vi "FFT.vi"() -> ()   [LabVIEW 2020]
uses:
  <vilib>/rvi/Analysis/measure/FFT/simModelSupport/niFPGA FFT Outside SCTL Sim Properties.ctl
  <vilib>/rvi/Analysis/measure/FFT/simModelSupport/niFPGA FFT Sim Types.ctl
  <vilib>/rvi/Analysis/measure/FFT/simModelSupport/niFpgaFFTSimArithmeticProperties.ctl
  <vilib>/rvi/Analysis/measure/FFT/simModelSupport/niFpgaFFTSimDfxp.ctl
  <vilib>/fxp/LVFixedPointQuantizationPolicyTypeDef.ctl
  <vilib>/rvi/Emulation/niFpgaGetClockAttributes.vi
  <vilib>/rvi/Emulation/niFpgaSctlEmulationGetInTimedLoop.vi
  <vilib>/rvi/Emulation/niFpgaEmulationReportErrorSimple.vi
  <vilib>/rvi/interface/RandomDataEmulation/niFpgaRandomDataHandleErrors.vi
  <vilib>/rvi/Analysis/measure/FFT/simModelSupport/niFpgaFFTSimModelOutsideSCTLCore.vi
  <vilib>/rvi/Emulation/niFpgaCriticalErrorInLSC.vi
  <vilib>/rvi/DataTransferAndStorage/Container/XNode/niFpgaContainer.xnode
  <vilib>/rvi/interface/RandomDataEmulation/nirviRandomDataFpgaReadWriteTemplate.vi
  <vilib>/rvi/Analysis/measure/FFT/XNode/niFpgaFFT.xnode
panel:
  out "x-y (microsecond)":u32
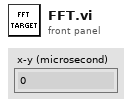
[diagram p1: front panel]
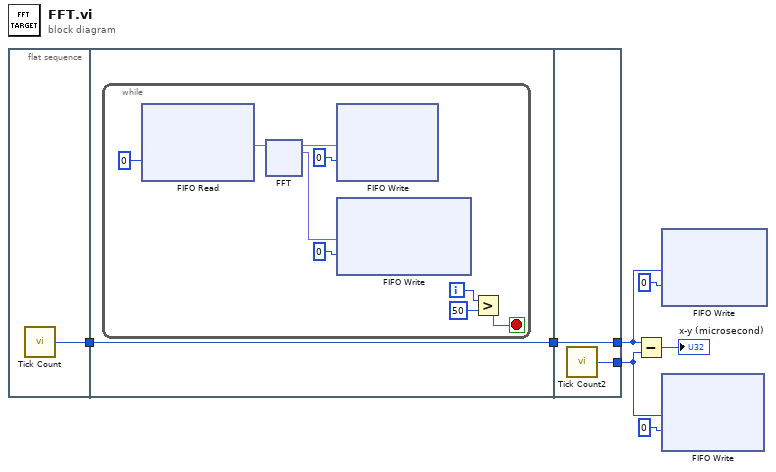
[diagram p0: block diagram]
diagram:
  n1 = flat-sequence {
    tunnel: [w8] -> w7
    tunnel: [w9] -> w6
    tunnel: w7 -> [w9]
    tunnel: [w40] -> w4
    tunnel: w6 -> [w40]
    tunnel: [w39] -> w3
    frame #0 {
      n2 = call "Tick Count"() -> ("Tick Count(uSec)"=w8:u32)
    }
    frame #1 {
      n3 = while {
        i -> [w17]
        stop <- w15 stop-if-true
        n4 = xnode ("FIFO Read")("Timeout"=0) -> ("Element"=w18:fxp<+/-,32,16>)  [unwired: 1 in, 2 out]
        n5 = xnode "FFT"("real data in"=w18) -> ("real data out"=w11:fxp<+/-,32,26>, "imaginary data out"=w10:fxp<+/-,32,26>)  [unwired: 2 in, 2 out]
        n6 = xnode ("FIFO Write")("Element"=w11, "Timeout"=0) -> ()  [unwired: 1 in, 2 out]
        n7 = xnode ("FIFO Write")("Element"=w10, "Timeout"=0) -> ()  [unwired: 1 in, 2 out]
        n8 = Greater?(x=w17, y=50) -> (0:w15:bool)
      }
    }
    frame #2 {
      n9 = call "Tick Count2"() -> ("Tick Count(uSec)"=w39:u32)
    }
  }
  n10 = Subtract(x=w4, y=w3) -> (x-y=→"x-y (microsecond)":u32)
  n11 = xnode ("FIFO Write")("Element"=w4, "Timeout"=0) -> ()  [unwired: 1 in, 2 out]
  n12 = xnode ("FIFO Write")("Element"=w3, "Timeout"=0) -> ()  [unwired: 1 in, 2 out]
